vi "Double FFT Mesurament (Control - Init Wave&Window - Snapshot - DoubleFFT - Latency - Low Freq - FREQ LIN) RT Test.vi"() -> ()   [LabVIEW 2014]
uses:
  <vilib>/Platform/TimedLoop/XDataNode/timing_clust.ctl
  <vilib>/Platform/TimedLoop/XDataNode/nitl_modes.ctl
  <vilib>/Platform/TimedLoop/XDataNode/wakeup.ctl
  <vilib>/FPGAPlugInAG/sbRIO-9636/niLvFpga_Open_sbRIO-9636.vi
  <vilib>/rvi/interface/common/dynamic/niFpgaDynamicAddResources.vi
  <vilib>/Utility/error.llb/Error Cluster From Error Code.vi
  <vilib>/rvi/errors/niLvFpgaAdjustHostInterfaceError.vi
  <vilib>/rvi/interface/common/niFpgaWaitOnOcc.vi
  <vilib>/FPGAPlugInAG/Dynamic/niLvFpga_Run_Dynamic.vi
  <vilib>/FPGAPlugInAG/Dynamic/niLvFpga_Abort_Dynamic.vi
  <vilib>/FPGAPlugInAG/Dynamic/niLvFpga_Reset_Dynamic.vi
  <vilib>/FPGAPlugInAG/Dynamic/niLvFpga_Close_Dynamic.vi
  <vilib>/rvi/interface/nirviOpenFPGA/nirviOpenFPGA.xnode
  FPGA Bitfiles/LaserDistanceSen_FPGATarget_DoubleFFTMesuram_744PzgZsl5A.lvbitx
  FPGA Target/Test VIs/Double FFT Mesurament (Control - Init Wave&Window - Snapshot - DoubleFFT - Latency - Low Freq) test.vi
  <vilib>/rvi/interface/nirviReadWriteControl/nirviReadWriteControl.xnode
  <vilib>/rvi/interface/nirviMethod/nirviMethod.xnode
  <vilib>/Platform/TimedLoop/XDataNode/XDataNode.xnode
  <vilib>/rvi/interface/nirviCloseFPGA/nirviCloseFPGA.xnode
  <vilib>/FPGAPlugInAG/Dynamic/niLvFpga_ConfigureFifo_Dynamic.vi
  <vilib>/rvi/errors/niLvFpgaMergeErrorWithErrorCode.vi
  <vilib>/FPGAPlugInAG/Dynamic/niLvFpga_StartFifo_Dynamic.vi
  <vilib>/rvi/interface/Simulation/niFpgaSimulationCallBeginRW.vi
  <vilib>/FPGAPlugInAG/Dynamic/niLvFpga_ReadFifo_Dynamic.vi
  <vilib>/Platform/TimedLoop/XDataNode/XDNodeRunTimeDep.lvlib
  NiFpgaLv.dll
panel:
  in  "Acrive  Smooth":bool=TRUE
  out "Complete SkewTri":dbl[](graph)
  out "2) Tri edge":dbl[](graph)
  out "1) Tri edge":dbl[](graph)
  out "1) Ext Mean Freq Curve":dbl[](graph)
  out "2) Ext Mean Freq Curve":dbl[](graph)
  out "2) Mean Freq Curve":dbl[](graph)
  out "1) Mean Freq Curve":dbl[](graph)
  out "2) Freq curve":dbl[](graph)
  out "1) Freq curve":dbl[](graph)
  in  "FFT Sliding Win Size":i32=128
  out "1) SmoothSubSig":dbl[](graph)
  out "2) SmoothSubSig":dbl[](graph)
  in  "Acrive Fit":bool=TRUE
  in  "Poly Order":i32=3
  in  "Side points":i32=13
  in  "Poly Grade":dbl=5.0
  out "2) Signal&Fit 2":dbl[][](graph)
  out "1) Signal&Fit":dbl[][](graph)
  in  "tieni premuto per":i32=1
  out "Current Sig lin":i32
  in  "Acrive Linearization":bool
  in  "# Measurements for Linearization":i32=10
  in  "stop":bool
  out "maxbin_secondFFT":i32
  out "maxbin_firstFFT":i32
  out "f_rise":dbl
  out "f_fall":dbl
  out "f_mean":dbl
  out "Velocity (m/s)":dbl
  out "Distance (m)":dbl
  in  "Initial Latency points":u32(slide)=28 scale=0.0..1249.0
  out "Second FFT (bin)":dbl[](graph)
  out "Second Signal (points) - Rising Triangular":dbl[](graph)
  out "First FFT (bin)":dbl[](graph)
  out "First Signal (points) - Falling Triangular":dbl[](graph)
  in  "Snapshot":bool
  in  "Windowing":T1(ring)
  in  "first bin":i32=5
  in  "last bin":i32=255
  in  "lower limit 2":u32(slide)=738 scale=625.0..738.0
  in  "lower limit 1":u32(slide)=113 scale=0.0..113.0
  # "WARNING:\nOnce pressed wait untill the end of operation"
  # "OFFLINE parameters"
  # "Max Detection FFT bin range"
  # "ONLINE parameters"
  # "Se la sottrazione del fondo non è eseguita su FPGA.\n Attivarla per eseguirla lato RT"
  # "Smoothing (S-G Params)"
  # "Fitting"
  # "ONLY POWER OF 2"
  # "Min: 2 Max: 256 (2, 4, 8, 16, 32, 64, 128, 256)"
  # "LINEARIZATION FINAL RESULTS"
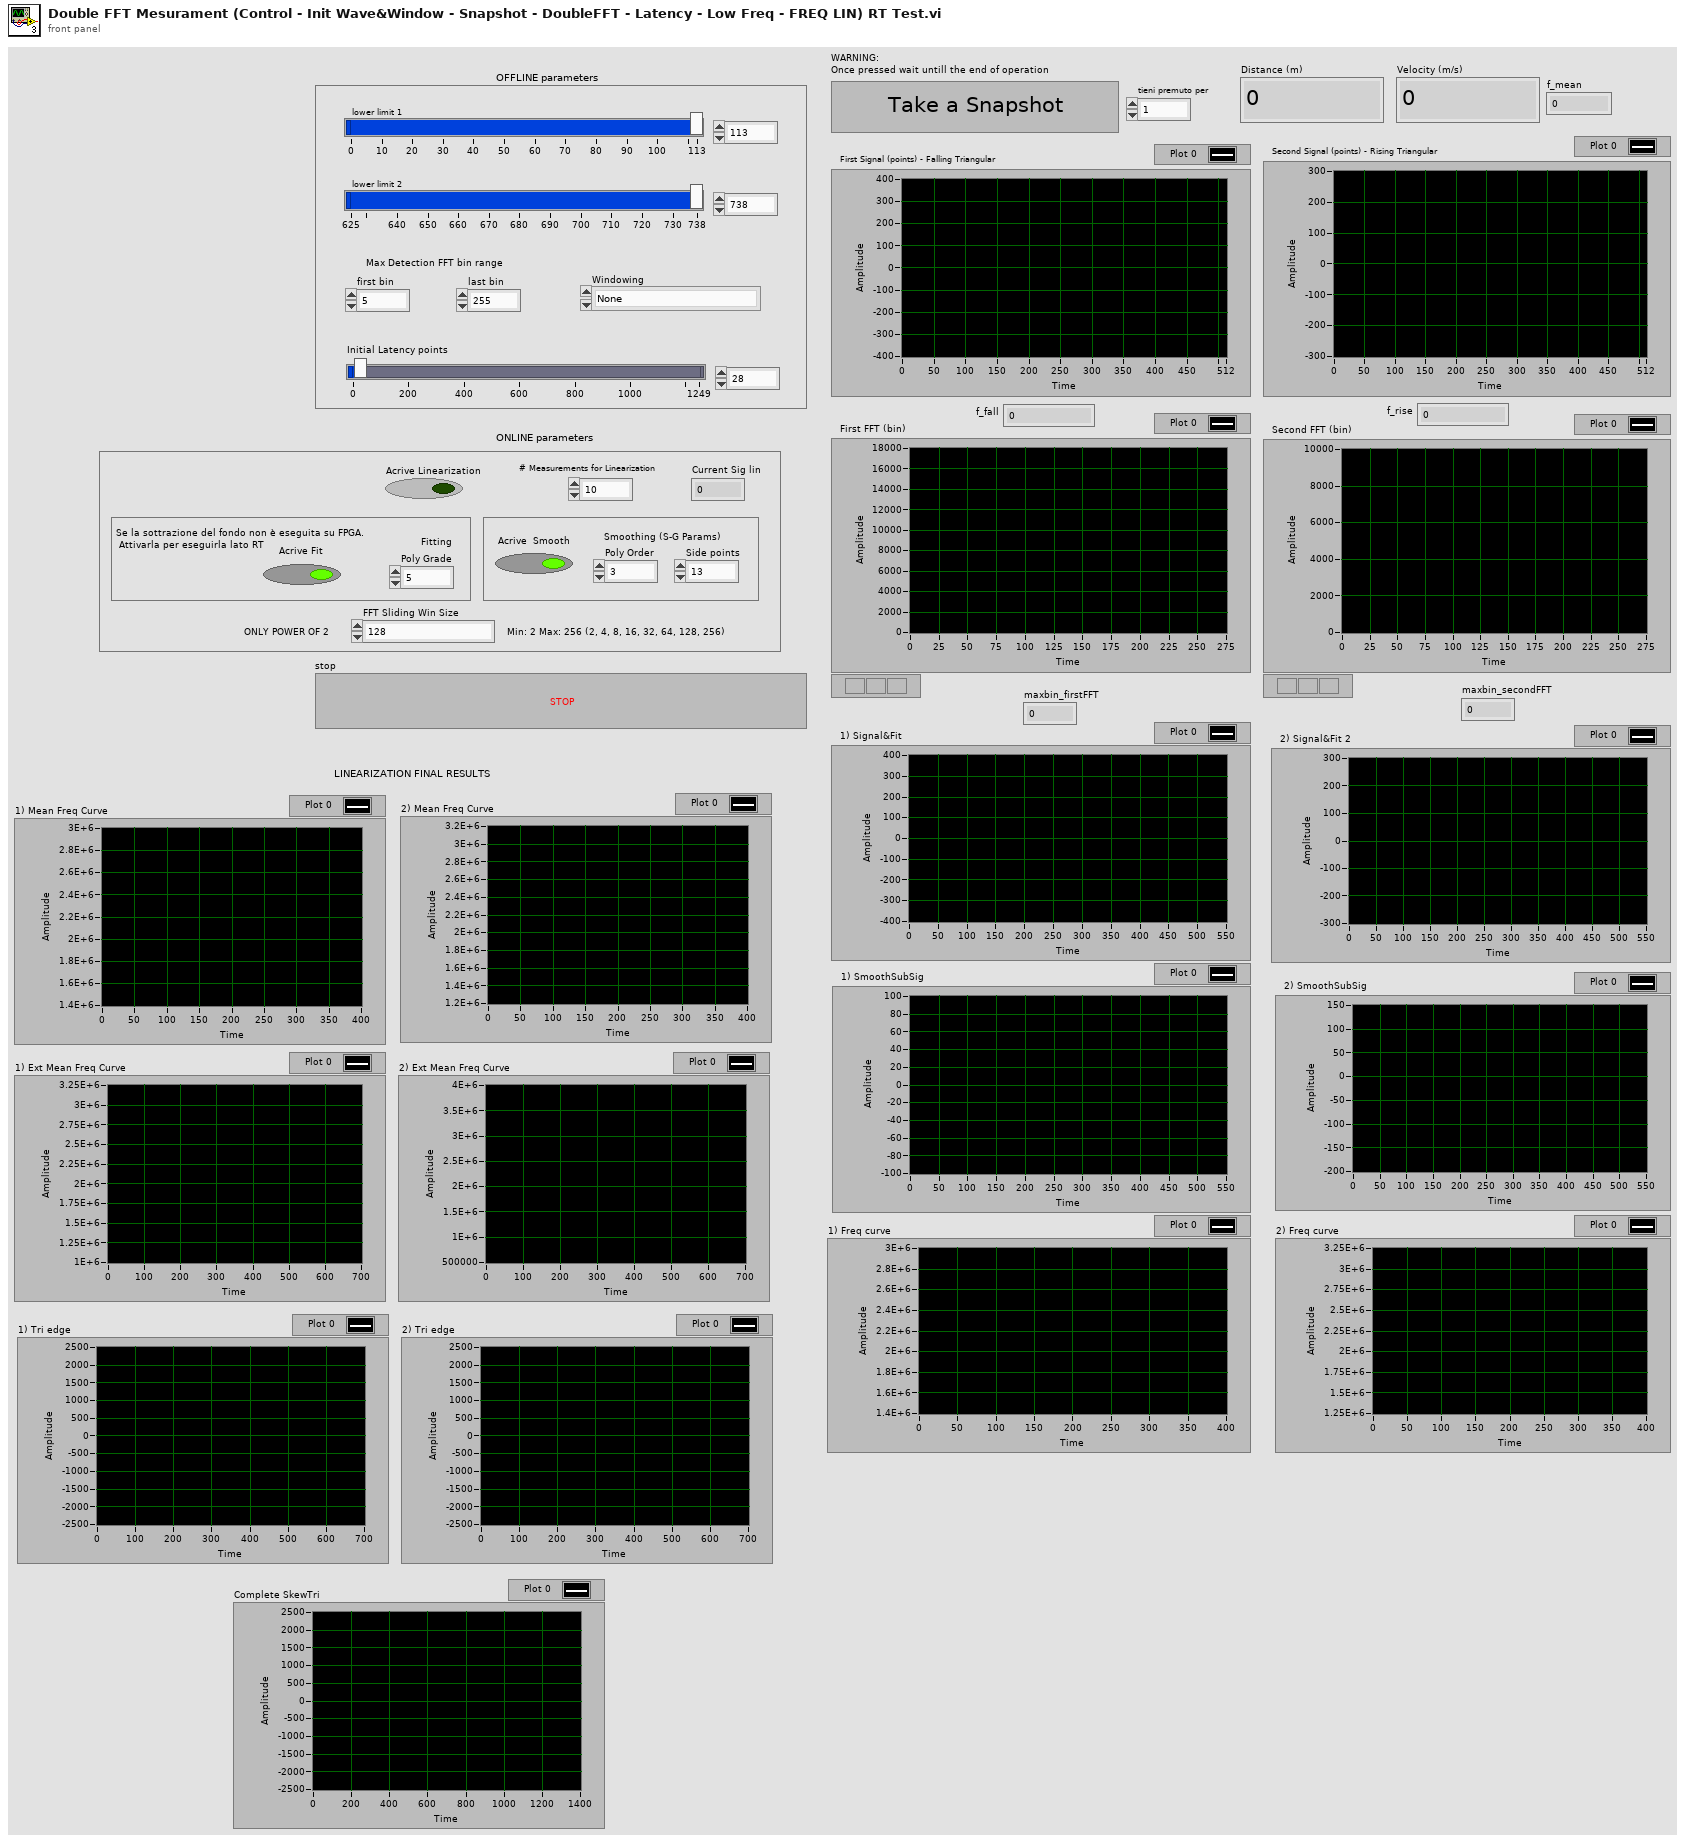
[diagram p1: front panel]
types:
  T1 = enum16{"None", "Hanning", "Hamming", "Blackman", "Blackman-Harris"}
  T2 = typedef "XDNodeRunTimeDep.lvlib/timing_clust.ctl" = cluster{"Expected End [f-1]":u64, "Actual End [f-1]":u64, "Finished Late? [f-1]":bool, "Expected End [i-1]":u64, "Actual End [i-1]":u64, "Finished Late? [i-1]":bool, "Expected Start [i]":u64, "Actual Start [i]":u64, "Expected Start [f]":u64, "Actual Start [f]":u64, "Source Name":string, "Structure Name":string, "Period":i64, "Deadline":i64, "Offset":i64, "Start":i64, "Priority":i32, "Timeout":i32, "Mode":T3, "Wakeup Reason":T4, "Error":errorcluster, "Source Type":string, "Secondary Source Type":string, "Global End Time":u64, "Global Start Time":u64, "Frame Duration":u64, "Iteration Duration":u64, "Assigned CPU":i32, "I/O Scan Engine Mode":u32}
  T3 = typedef "XDNodeRunTimeDep.lvlib/nitl_modes.ctl" = enum32{"No Change", "Process missed periods, maintain original phase", "Discard missed periods, maintain original phase", "Process missed periods, ignore original phase", "Discard missed periods, ignore original phase"}
  T4 = typedef "XDNodeRunTimeDep.lvlib/wakeup.ctl" = enum32{"Normal", "Aborted", "Asynchronous wakeup", "Timing source error", "Timed loop error", "Timeout"}
  T5 = typedef "NI_Matrix.lvlib/RealMatrix.ctl" = dbl[][]
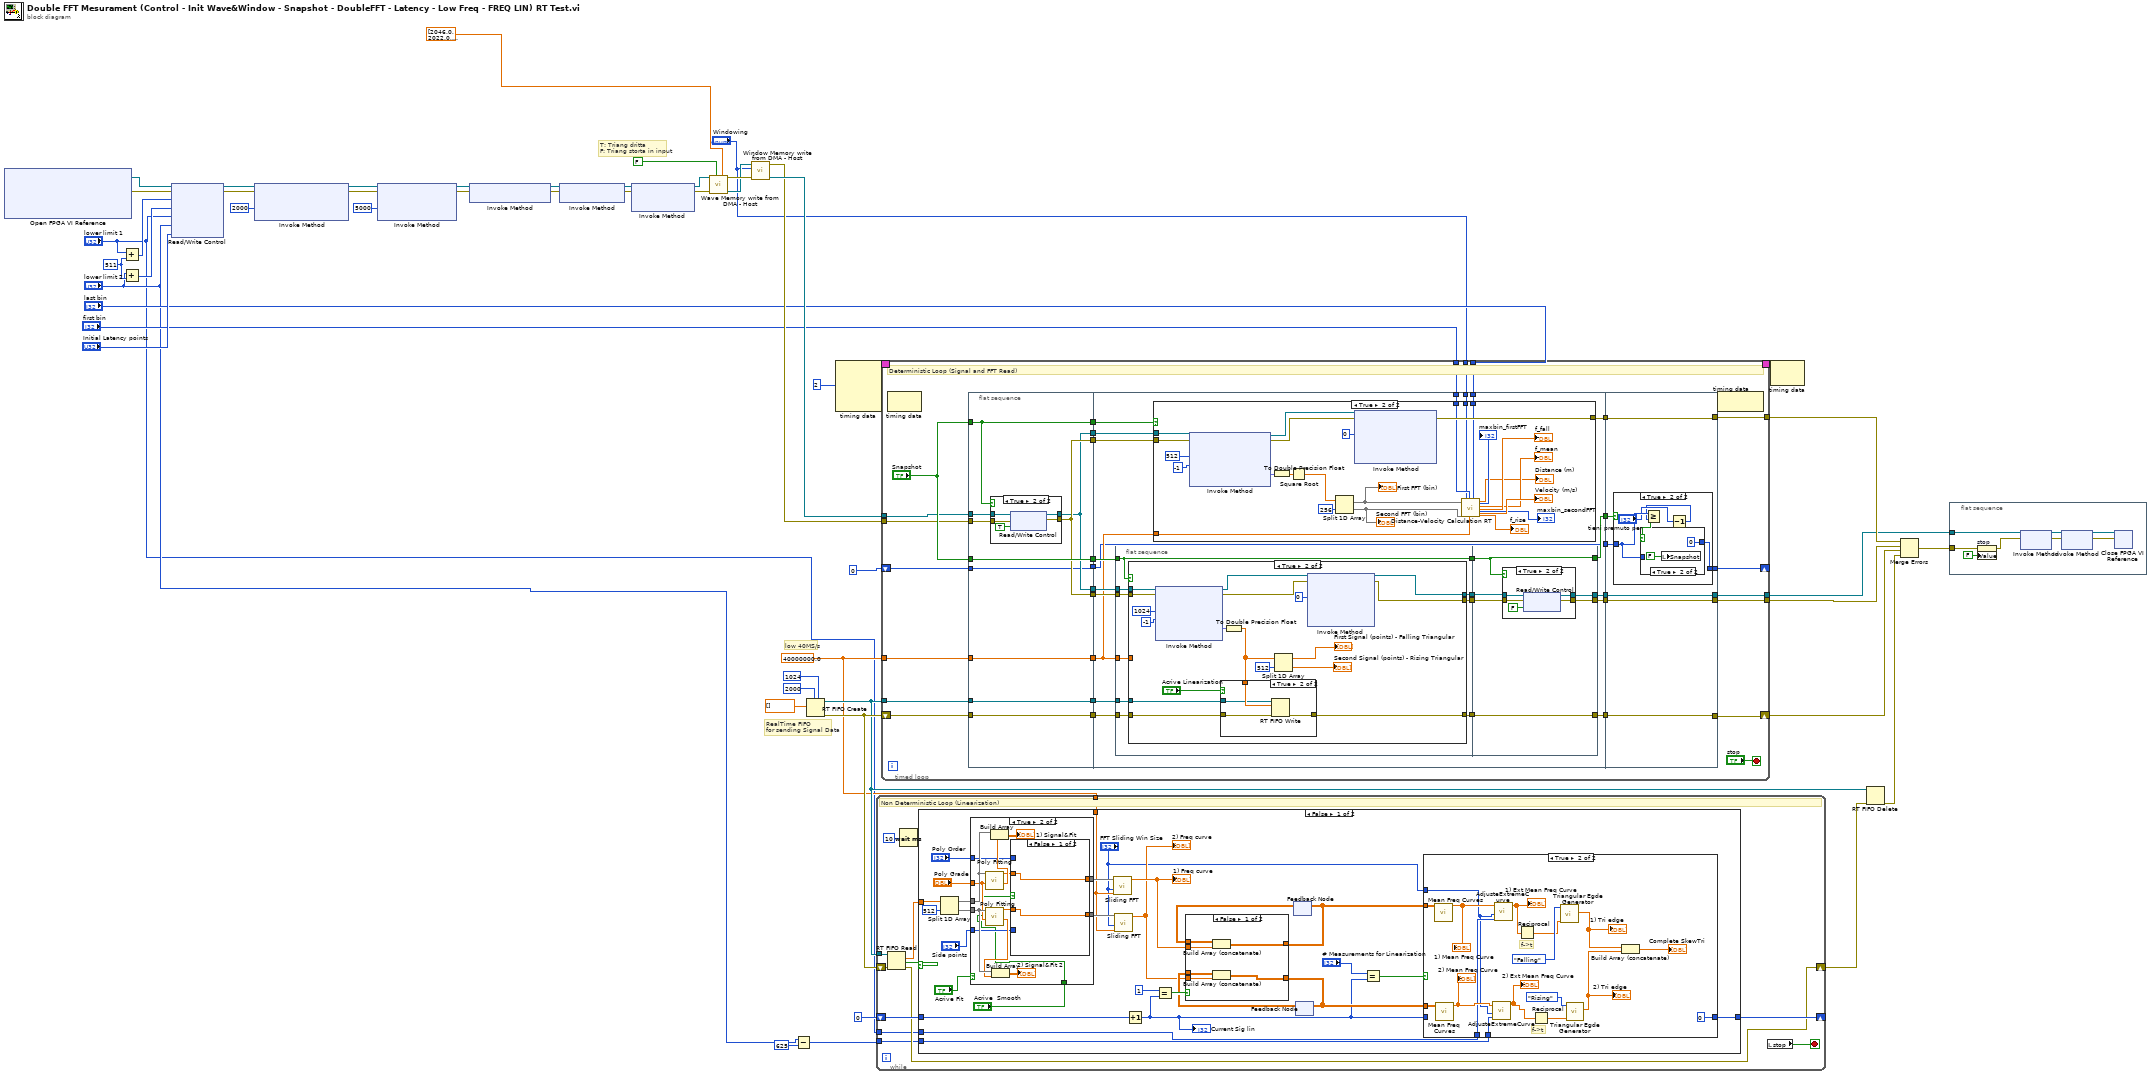
[diagram p0: block diagram]
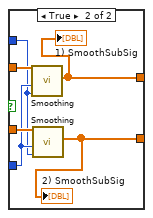
[diagram p3: hidden frame]
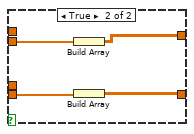
[diagram p5: hidden frame]
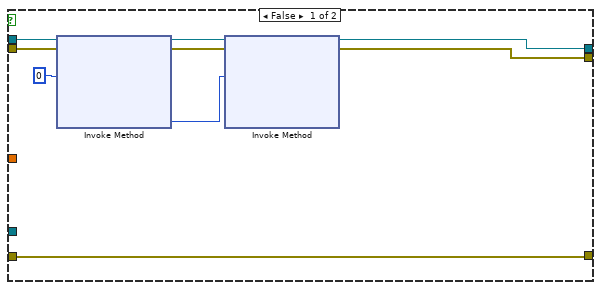
[diagram p8: hidden frame]
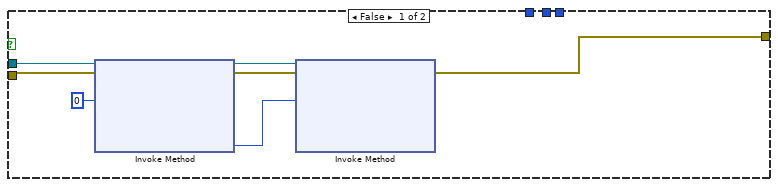
[diagram p11: hidden frame]
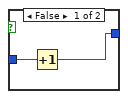
[diagram p13: hidden frame]
diagram:
  w49 = u32 511 ("y")
  w4 = 40000000.0 ("Sample Rate (S/s)")
  # "T: Triang dritta\nF: Triang storta in input"
  # "RealTime FIFO \nfor sending Signal Data"
  # "low 40MS/s"
  n1 = xnode "Open FPGA VI Reference"() -> ("FPGA VI Reference Out"=w48:refnum<k20>, "error out"=w47:errorcluster)  [unwired: 2 in]
  n2 = Add(x="lower limit 1", y=w49) -> (x+y=w51:u32)
  n3 = Add(x="lower limit 2", y=w49) -> (x+y=w50:u32)
  n4 = xnode "Read/Write Control"("FPGA VI Reference In"=w48, "error in"=w47, "upper limit 1"=w51, "upper limit 2"=w50, "lower limit 1"="lower limit 1", "lower limit 2"="lower limit 2", "Latency points"="Initial Latency points") -> ("FPGA VI Reference Out"=w44:refnum<k20>, "error out"=w43:errorcluster)
  n5 = xnode "Invoke Method"("FPGA VI Reference In"=w44, "error in"=w43, "Requested Depth"=u32 2000) -> ("FPGA VI Reference Out"=w22:refnum<k20>, "error out"=w23:errorcluster)  [unwired: 1 out]
  n6 = xnode "Invoke Method"("FPGA VI Reference In"=w22, "error in"=w23, "Requested Depth"=u32 5000) -> ("FPGA VI Reference Out"=w36:refnum<k20>, "error out"=w37:errorcluster)  [unwired: 1 out]
  n7 = xnode "Invoke Method"("FPGA VI Reference In"=w36, "error in"=w37) -> ("FPGA VI Reference Out"=w20:refnum<k20>, "error out"=w21:errorcluster)
  n8 = xnode "Invoke Method"("FPGA VI Reference In"=w20, "error in"=w21) -> ("FPGA VI Reference Out"=w34:refnum<k20>, "error out"=w35:errorcluster)
  n9 = xnode "Invoke Method"("FPGA VI Reference In"=w34, "error in"=w35) -> ("FPGA VI Reference Out"=w40:refnum<k20>, "error out"=w39:errorcluster)  [unwired: 1 in]
  n10 = call "Wave Memory write from DMA - Host.vi"("Custom Triangular Signal (fal-ris)"=dbl[] [2046.0, 2022.0, 1999.0, 1975.0, 1952.0, 1928.0, 1905.0, 1882.0, 1860.0, 1837.0, 1815.0, 1793.0, 1771.0, 1749.0, 1728.0, 1706.0, 1685.0, 1664.0, 1643.0, 1622.0, 1602.0, 1581.0, 1561.0, 1541.0, 1521.0, 1501.0, 1482.0, 1462.0, 1443.0, 1424.0, 1405.0, 1386.0, 1367.0, 1348.0, 1330.0, 1312.0, 1293.0, 1275.0, 1257.0, 1240.0, 1222.0, 1204.0, 1187.0, 1170.0, 1153.0, 1136.0, 1119.0, 1102.0, 1085.0, 1069.0, 1052.0, 1036.0, 1020.0, 1004.0, 988.0, 972.0, 956.0, 940.0, 925.0, 910.0, 894.0, 879.0, 864.0, 849.0, 834.0, 819.0, 804.0, 790.0, 775.0, 761.0, 747.0, 732.0, 718.0, 704.0, 690.0, 676.0, 663.0, 649.0, 635.0, 622.0, 608.0, 595.0, 582.0, 569.0, 555.0, 542.0, 530.0, 517.0, 504.0, 491.0, 479.0, 466.0, 454.0, 441.0, 429.0, 417.0, 405.0, 393.0, 381.0, 369.0, 357.0, 345.0, 333.0, 322.0, 310.0, 299.0, 287.0, 276.0, 265.0, 253.0, 242.0, 231.0, 220.0, 209.0, 198.0, 187.0, 176.0, 166.0, 155.0, 144.0, 134.0, 123.0, 113.0, 103.0, 92.0, 82.0, 72.0, 62.0, 52.0, 42.0, 32.0, 22.0, 12.0, 2.0, -8.0, -17.0, -27.0, -37.0, -46.0, -56.0, -65.0, -75.0, -84.0, -93.0, -102.0, -112.0, -121.0, -130.0, -139.0, -148.0, -157.0, -166.0, -175.0, -184.0, -192.0, -201.0, -210.0, -218.0, -227.0, -235.0, -244.0, -252.0, -261.0, -269.0, -278.0, -289.0, -298.0, -306.0, -314.0, -323.0, -331.0, -339.0, -348.0, -356.0, -364.0, -372.0, -380.0, -388.0, -396.0, -404.0, -412.0, -420.0, -428.0, -436.0, -443.0, -451.0, -458.0, -466.0, -473.0, -481.0, -488.0, -495.0, -502.0, -509.0, -516.0, -523.0, -530.0, -536.0, -543.0, -550.0, -562.0, -568.0, -575.0, -587.0, -595.0, -602.0, -608.0, -614.0, -621.0, -627.0, -637.0, -643.0, -650.0, -656.0, -666.0, -672.0, -681.0, -689.0, -696.0, -702.0, -707.0, -713.0, -719.0, -725.0, -730.0, -736.0, -742.0, -747.0, -753.0, -758.0, -764.0, -769.0, -775.0, -780.0, -786.0, -791.0, -797.0, -802.0, -807.0, -813.0, -818.0, -823.0, -828.0, -833.0, -839.0, -844.0, -849.0, -854.0, -859.0, -864.0, -870.0, -875.0, -880.0, -885.0, -890.0, -895.0, -900.0, -905.0, -910.0, -915.0, -919.0, -924.0, -929.0, -934.0, -940.0, -945.0, -950.0, -954.0, -959.0, -964.0, -969.0, -974.0, -978.0, -984.0, -989.0, -994.0, -1000.0, -1004.0, -1009.0, -1013.0, -1019.0, -1023.0, -1027.0, -1032.0, -1037.0, -1042.0, -1047.0, -1052.0, -1056.0, -1060.0, -1065.0, -1069.0, -1073.0, -1077.0, -1081.0, -1085.0, -1089.0, -1093.0, -1097.0, -1101.0, -1105.0, -1109.0, -1113.0, -1116.0, -1120.0, -1124.0, -1128.0, -1131.0, -1135.0, -1139.0, -1142.0, -1146.0, -1150.0, -1153.0, -1157.0, -1161.0, -1164.0, -1168.0, -1171.0, -1175.0, -1178.0, -1182.0, -1185.0, -1189.0, -1192.0, -1196.0, -1199.0, -1203.0, -1206.0, -1210.0, -1213.0, -1217.0, -1220.0, -1224.0, -1227.0, -1231.0, -1234.0, -1237.0, -1241.0, -1244.0, -1248.0, -1251.0, -1255.0, -1258.0, -1262.0, -1265.0, -1268.0, -1272.0, -1275.0, -1279.0, -1282.0, -1286.0, -1289.0, -1292.0, -1296.0, -1299.0, -1303.0, -1306.0, -1310.0, -1313.0, -1316.0, -1320.0, -1323.0, -1327.0, -1330.0, -1334.0, -1337.0, -1340.0, -1344.0, -1347.0, -1351.0, -1354.0, -1357.0, -1361.0, -1364.0, -1368.0, -1371.0, -1374.0, -1377.0, -1381.0, -1384.0, -1387.0, -1390.0, -1394.0, -1397.0, -1400.0, -1404.0, -1407.0, -1410.0, -1413.0, -1417.0, -1420.0, -1423.0, -1426.0, -1429.0, -1432.0, -1435.0, -1438.0, -1441.0, -1444.0, -1448.0, -1451.0, -1454.0, -1457.0, -1460.0, -1463.0, -1466.0, -1469.0, -1472.0, -1475.0, -1478.0, -1481.0, -1484.0, -1487.0, -1490.0, -1493.0, -1496.0, -1499.0, -1502.0, -1505.0, -1508.0, -1511.0, -1515.0, -1517.0, -1520.0, -1523.0, -1526.0, -1529.0, -1533.0, -1536.0, -1539.0, -1542.0, -1544.0, -1547.0, -1550.0, -1553.0, -1556.0, -1559.0, -1562.0, -1565.0, -1568.0, -1570.0, -1573.0, -1576.0, -1579.0, -1582.0, -1585.0, -1587.0, -1590.0, -1593.0, -1596.0, -1599.0, -1602.0, -1604.0, -1607.0, -1610.0, -1613.0, -1616.0, -1618.0, -1621.0, -1624.0, -1627.0, -1630.0, -1632.0, -1635.0, -1638.0, -1641.0, -1644.0, -1646.0, -1649.0, -1652.0, -1655.0, -1657.0, -1660.0, -1663.0, -1666.0, -1668.0, -1671.0, -1674.0, -1677.0, -1679.0, -1682.0, -1685.0, -1688.0, -1690.0, -1693.0, -1696.0, -1699.0, -1701.0, -1704.0, -1707.0, -1709.0, -1712.0, -1715.0, -1718.0, -1720.0, -1723.0, -1726.0, -1728.0, -1731.0, -1734.0, -1736.0, -1739.0, -1742.0, -1744.0, -1747.0, -1750.0, -1752.0, -1755.0, -1758.0, -1760.0, -1763.0, -1766.0, -1768.0, -1771.0, -1774.0, -1776.0, -1779.0, -1782.0, -1784.0, -1787.0, -1790.0, -1792.0, -1795.0, -1797.0, -1800.0, -1803.0, -1805.0, -1808.0, -1811.0, -1813.0, -1816.0, -1818.0, -1821.0, -1824.0, -1826.0, -1829.0, -1831.0, -1834.0, -1837.0, -1839.0, -1842.0, -1844.0, -1847.0, -1850.0, -1852.0, -1855.0, -1857.0, -1860.0, -1862.0, -1865.0, -1868.0, -1870.0, -1873.0, -1875.0, -1878.0, -1880.0, -1883.0, -1885.0, -1888.0, -1891.0, -1893.0, -1896.0, -1898.0, -1901.0, -1903.0, -1906.0, -1908.0, -1911.0, -1913.0, -1916.0, -1918.0, -1921.0, -1923.0, -1926.0, -1928.0, -1931.0, -1933.0, -1936.0, -1938.0, -1941.0, -1943.0, -1946.0, -1948.0, -1951.0, -1953.0, -1956.0, -1958.0, -1961.0, -1963.0, -1966.0, -1968.0, -1971.0, -1973.0, -1976.0, -1978.0, -1981.0, -1983.0, -1985.0, -1988.0, -1990.0, -1993.0, -1995.0, -1998.0, -2000.0, -2003.0, -2005.0, -2007.0, -2010.0, -2012.0, -2015.0, -2017.0, -2020.0, -2022.0, -2024.0, -2027.0, -2029.0, -2032.0, -2034.0, -2036.0, -2039.0, -2041.0, -2044.0, -2046.0, -2048.0, -2048.0, -2013.0, -1979.0, -1945.0, -1911.0, -1879.0, -1847.0, -1815.0, -1784.0, -1754.0, -1724.0, -1694.0, -1666.0, -1637.0, -1609.0, -1582.0, -1555.0, -1529.0, -1503.0, -1477.0, -1452.0, -1427.0, -1403.0, -1379.0, -1355.0, -1332.0, -1309.0, -1286.0, -1264.0, -1242.0, -1221.0, -1200.0, -1179.0, -1158.0, -1138.0, -1118.0, -1098.0, -1079.0, -1060.0, -1041.0, -1022.0, -1004.0, -986.0, -968.0, -950.0, -933.0, -916.0, -899.0, -882.0, -866.0, -849.0, -833.0, -818.0, -802.0, -786.0, -771.0, -756.0, -741.0, -727.0, -712.0, -698.0, -684.0, -670.0, -656.0, -642.0, -629.0, -616.0, -602.0, -589.0, -576.0, -564.0, -551.0, -539.0, -527.0, -514.0, -502.0, -491.0, -479.0, -467.0, -456.0, -444.0, -433.0, -422.0, -411.0, -400.0, -389.0, -379.0, -368.0, -358.0, -348.0, -337.0, -327.0, -317.0, -307.0, -298.0, -288.0, -278.0, -269.0, -259.0, -250.0, -241.0, -232.0, -223.0, -214.0, -205.0, -196.0, -187.0, -179.0, -170.0, -162.0, -154.0, -145.0, -137.0, -129.0, -121.0, -113.0, -105.0, -97.0, -89.0, -82.0, -74.0, -66.0, -59.0, -51.0, -44.0, -37.0, -30.0, -22.0, -15.0, -8.0, -1.0, 6.0, 13.0, 19.0, 26.0, 33.0, 40.0, 46.0, 53.0, 59.0, 66.0, 72.0, 78.0, 85.0, 91.0, 97.0, 103.0, 109.0, 115.0, 121.0, 127.0, 133.0, 139.0, 145.0, 150.0, 156.0, 162.0, 167.0, 173.0, 178.0, 184.0, 189.0, 195.0, 200.0, 205.0, 211.0, 216.0, 221.0, 226.0, 231.0, 232.0, 238.0, 243.0, 249.0, 254.0, 259.0, 265.0, 270.0, 276.0, 281.0, 281.0, 283.0, 289.0, 294.0, 288.0, 273.0, 276.0, 282.0, 288.0, 293.0, 296.0, 293.0, 295.0, 301.0, 307.0, 313.0, 309.0, 314.0, 314.0, 314.0, 319.0, 324.0, 328.0, 333.0, 338.0, 342.0, 347.0, 351.0, 356.0, 360.0, 365.0, 369.0, 374.0, 378.0, 383.0, 387.0, 392.0, 396.0, 401.0, 402.0, 407.0, 412.0, 413.0, 418.0, 424.0, 429.0, 431.0, 437.0, 443.0, 448.0, 447.0, 448.0, 451.0, 455.0, 461.0, 464.0, 459.0, 465.0, 470.0, 474.0, 480.0, 484.0, 490.0, 490.0, 496.0, 502.0, 508.0, 513.0, 519.0, 525.0, 530.0, 536.0, 536.0, 541.0, 547.0, 552.0, 558.0, 563.0, 569.0, 574.0, 579.0, 584.0, 590.0, 595.0, 600.0, 605.0, 611.0, 616.0, 621.0, 627.0, 632.0, 637.0, 642.0, 648.0, 653.0, 659.0, 664.0, 669.0, 675.0, 680.0, 686.0, 691.0, 697.0, 702.0, 708.0, 714.0, 719.0, 725.0, 725.0, 731.0, 737.0, 744.0, 747.0, 753.0, 759.0, 766.0, 772.0, 777.0, 784.0, 790.0, 798.0, 805.0, 811.0, 816.0, 815.0, 821.0, 823.0, 826.0, 831.0, 837.0, 842.0, 840.0, 843.0, 845.0, 851.0, 856.0, 861.0, 866.0, 871.0, 869.0, 869.0, 873.0, 878.0, 883.0, 887.0, 892.0, 897.0, 901.0, 906.0, 906.0, 910.0, 914.0, 918.0, 922.0, 926.0, 930.0, 934.0, 937.0, 941.0, 945.0, 949.0, 953.0, 956.0, 960.0, 964.0, 968.0, 972.0, 976.0, 980.0, 984.0, 988.0, 992.0, 996.0, 1000.0, 1004.0, 1008.0, 1012.0, 1016.0, 1021.0, 1026.0, 1031.0, 1036.0, 1041.0, 1045.0, 1050.0, 1055.0, 1054.0, 1059.0, 1061.0, 1060.0, 1065.0, 1070.0, 1075.0, 1080.0, 1083.0, 1086.0, 1091.0, 1094.0, 1097.0, 1098.0, 1101.0, 1105.0, 1110.0, 1113.0, 1117.0, 1122.0, 1126.0, 1131.0, 1136.0, 1139.0, 1144.0, 1148.0, 1153.0, 1158.0, 1163.0, 1167.0, 1172.0, 1177.0, 1182.0, 1186.0, 1191.0, 1196.0, 1201.0, 1206.0, 1210.0, 1215.0, 1220.0, 1225.0, 1230.0, 1235.0, 1240.0, 1245.0, 1250.0, 1255.0, 1260.0, 1265.0, 1270.0, 1275.0, 1280.0, 1285.0, 1290.0, 1295.0, 1301.0, 1306.0, 1311.0, 1316.0, 1321.0, 1326.0, 1331.0, 1335.0, 1340.0, 1345.0, 1350.0, 1355.0, 1359.0, 1364.0, 1369.0, 1373.0, 1378.0, 1382.0, 1387.0, 1391.0, 1396.0, 1400.0, 1404.0, 1408.0, 1413.0, 1417.0, 1421.0, 1425.0, 1429.0, 1434.0, 1438.0, 1442.0, 1446.0, 1450.0, 1454.0, 1459.0, 1463.0, 1467.0, 1471.0, 1475.0, 1479.0, 1483.0, 1487.0, 1491.0, 1495.0, 1499.0, 1503.0, 1507.0, 1511.0, 1515.0, 1519.0, 1523.0, 1527.0, 1531.0, 1535.0, 1539.0, 1543.0, 1547.0, 1551.0, 1555.0, 1559.0, 1563.0, 1567.0, 1571.0, 1574.0, 1578.0, 1582.0, 1586.0, 1590.0, 1594.0, 1598.0, 1602.0, 1605.0, 1609.0, 1613.0, 1617.0, 1621.0, 1624.0, 1628.0, 1632.0, 1636.0, 1639.0, 1643.0, 1647.0, 1651.0, 1654.0, 1658.0, 1662.0, 1666.0, 1669.0, 1673.0, 1677.0, 1680.0, 1684.0, 1688.0, 1691.0, 1695.0, 1699.0, 1702.0, 1706.0, 1710.0, 1713.0, 1717.0, 1720.0, 1724.0, 1728.0, 1731.0, 1735.0, 1738.0, 1742.0, 1745.0, 1749.0, 1753.0, 1756.0, 1760.0, 1763.0, 1767.0, 1770.0, 1774.0, 1777.0, 1781.0, 1784.0, 1788.0, 1791.0, 1795.0, 1798.0, 1802.0, 1805.0, 1808.0, 1812.0, 1815.0, 1819.0, 1822.0, 1826.0, 1829.0, 1832.0, 1836.0, 1839.0, 1842.0, 1846.0, 1849.0, 1853.0, 1856.0, 1859.0, 1863.0, 1866.0, 1869.0, 1873.0, 1876.0, 1879.0, 1883.0, 1886.0, 1889.0, 1892.0, 1896.0, 1899.0, 1902.0, 1906.0, 1909.0, 1912.0, 1915.0, 1918.0, 1922.0, 1925.0, 1928.0, 1931.0, 1935.0, 1938.0, 1941.0, 1944.0, 1947.0, 1951.0, 1954.0, 1957.0, 1960.0, 1963.0, 1966.0, 1970.0, 1973.0, 1976.0, 1979.0, 1982.0, 1985.0, 1988.0, 1991.0, 1995.0, 1998.0, 2001.0, 2004.0, 2007.0, 2010.0, 2013.0, 2016.0, 2019.0, 2022.0, 2025.0, 2028.0, 2031.0, 2034.0, 2037.0, 2040.0, 2043.0, 2047.0] ("Complete SkewTri"), "Triangolo dritto?"=FALSE, "error in"=w39, "FPGA VI Reference In"=w40) -> ("FPGA VI Reference Out"=w25:refnum<k20>, "error out"=w38:errorcluster)  [unwired: 5 in, 1 out]
  n11 = call "Window Memory write from DMA - Host.vi"("error in"=w38, "Enum"="Windowing", "FPGA VI Reference In"=w25) -> ("FPGA VI Reference Out"=w46:refnum<k20>, "error out"=w45:errorcluster)  [unwired: 5 in, 2 out]
  n12 = Subtract(x="lower limit 2", y=u32 625) -> (x-y=w6:u32)
  n13 = RT FIFO Create(1:dbl[] [] ("double precision float"), 4:u32 2000 ("size (10)"), 6:u32 1024 ("elements in array (1)")) -> (8:w12:refnum<k33>, 11:w14:errorcluster)  [unwired: 5 in, 1 out]
  n14 = node-c288(i64 2 ("Period")) -> (w33:T2)  [unwired: 3 in]
  n15 = while {
    shift-right: [w55] -> w11
    shift-left: w14 -> [w57]
    tunnel: w12 -> [w62]
    shift-right: [w56] -> _
    shift-left: 0 -> [w60]
    tunnel: "lower limit 1" -> [w52]
    tunnel: w6 -> [w53]
    tunnel: w4 -> [w54]
    stop <- w61 stop-if-true
    # "Non Deterministic Loop (Linearization)"
    n16 = RT FIFO Read(0:w62, 3:w57) -> (9:w59:dbl[], 10:w58:bool, 11:w55:errorcluster)  [unwired: 2 in, 2 out]
    n17 = Wait (ms)(milliseconds to wait=u32 10 ("millisecond multiple")) -> ()  [unwired: 1 out]
    n18 = case shown="False" w58 {
      tunnel: w60 -> [w91 w144]
      tunnel: [w80 w144] -> w56
      tunnel: w59 -> [w89 _]
      tunnel: w54 -> [w70 _]
      tunnel: w53 -> [w67 _]
      tunnel: w52 -> [w66 _]
      frame False {
        n19 = Split 1D Array(array=w89, index=512) -> (first subarray=w78:dbl[], second subarray=w77:dbl[])
        n20 = case shown="True" "Acrive Fit" {
          tunnel: w78 -> [w93 w107]
          tunnel: w77 -> [w92 w103]
          tunnel: "Poly Grade" -> [_ w99]
          tunnel: "Side points" -> [_ w98]
          tunnel: "Poly Order" -> [_ w97]
          tunnel: [w92 w96] -> w71
          tunnel: [w93 w94] -> w72
          tunnel: "Acrive  Smooth" -> [_ w95]
          frame False {
          }
          frame True {
            n21 = call "Poly Fitting.vi"("Poly Grade"=w99, "Signal"=w107) -> ("Poly Signal"=w106:dbl[], "SubtractedSignal"=w101:dbl[])  [unwired: 8 in]
            n22 = call "Poly Fitting.vi"("Poly Grade"=w99, "Signal"=w103) -> ("Poly Signal"=w102:dbl[], "SubtractedSignal"=w100:dbl[])  [unwired: 8 in]
            n23 = Build Array(w107, w106) -> (→"1) Signal&Fit":dbl[][])
            n24 = Build Array(w103, w102) -> (→"2) Signal&Fit 2":dbl[][])
            n25 = case shown="False" w95 {
              tunnel: w101 -> [w109 w115]
              tunnel: w100 -> [w108 w114]
              tunnel: w98 -> [_ w113]
              tunnel: w97 -> [_ w112]
              tunnel: [w108 w111] -> w96
              tunnel: [w109 w110] -> w94
              frame False {
              }
              frame True {
                n26 = call "Smoothing.vi"("polynomial order"=w112, "side points"=w113, "SubtractedSignal"=w115) -> ("SubSmoothSignal"=w110:dbl[])  [unwired: 8 in]
                "1) SmoothSubSig" <- w110
                n27 = call "Smoothing.vi"("polynomial order"=w112, "side points"=w113, "SubtractedSignal"=w114) -> ("SubSmoothSignal"=w111:dbl[])  [unwired: 8 in]
                "2) SmoothSubSig" <- w111
              }
            }
          }
        }
        n28 = call "Sliding FFT.vi"("Sample Freq"=w70, "FFT Win Size"="FFT Sliding Win Size", "SubSmoothSignal"=w72) -> ("Freq samples"=w69:dbl[])  [unwired: 7 in, 1 out]
        "1) Freq curve" <- w69
        n29 = call "Sliding FFT.vi"("Sample Freq"=w70, "FFT Win Size"="FFT Sliding Win Size", "SubSmoothSignal"=w71) -> ("Freq samples"=w68:dbl[])  [unwired: 7 in, 1 out]
        "2) Freq curve" <- w68
        n30 = Increment(x=w91) -> (x+1=w81:i32)
        "Current Sig lin" <- w81
        n31 = Equal?(x=1, y=w81) -> (x = y?=w87:bool)
        n32 = feedback #1() -> (w86:T5)  [unwired: 1 in]
        n33 = feedback #2() -> (w85:T5)  [unwired: 1 in]
        n34 = case shown="False" w87 {
          tunnel: w68 -> [w138 w141]
          tunnel: w69 -> [w139 w143]
          tunnel: [w137 w140] -> w82
          tunnel: [w136 w142] -> w83
          tunnel: w86 -> [w135 _]
          tunnel: w85 -> [w134 _]
          frame False {
            n35 = Build Array (concatenate)(w135, w139) -> (w136:T5)
            n36 = Build Array (concatenate)(w134, w138) -> (w137:T5)
          }
          frame True {
            n37 = Build Array(w143) -> (w142:T5)
            n38 = Build Array(w141) -> (w140:T5)
          }
        }
        n39 = feedback-in #1(w83) -> ()
        n40 = feedback-in #2(w82) -> ()
        n41 = Equal?(x="# Measurements for Linearization", y=w81) -> (x = y?=w79:bool)
        n42 = case shown="True" w79 {
          tunnel: w83 -> [_ w132]
          tunnel: w82 -> [_ w131]
          tunnel: w81 -> [w116 _]
          tunnel: [w116 0] -> w80
          tunnel: w67 -> [_ w122]
          tunnel: w66 -> [_ w119]
          tunnel: "FFT Sliding Win Size" -> [_ w118]
          frame False {
          }
          frame True {
            # "f->t"
            # "f->t"
            n43 = call "Mean Freq Curves.vi"("Set of Freq samples"=w132) -> ("Mean Freq Curve"=w123:dbl[])  [unwired: 10 in]
            "1) Mean Freq Curve" <- w123
            n44 = call "Mean Freq Curves.vi"("Set of Freq samples"=w131) -> ("Mean Freq Curve"=w120:dbl[])  [unwired: 10 in]
            "2) Mean Freq Curve" <- w120
            n45 = call "AdjusteExtremeCurve.vi"("Init Bins Discarded"=w122, "FFT Size Window"=w118, "Freq sample"=w120) -> ("Extended Freq Sample"=w121:dbl[])  [unwired: 8 in]
            "2) Ext Mean Freq Curve" <- w121
            n46 = call "AdjusteExtremeCurve.vi"("Init Bins Discarded"=w119, "FFT Size Window"=w118, "Freq sample"=w123) -> ("Extended Freq Sample"=w117:dbl[])  [unwired: 8 in]
            "1) Ext Mean Freq Curve" <- w117
            n47 = Reciprocal(x=w117) -> (1/x=w125:dbl[])
            n48 = Reciprocal(x=w121) -> (1/x=w124:dbl[])
            n49 = call "Triangular Egde Generator.vi"("Sample values"=w125, "Triangular edge"=enum16{"Rising", "Falling"}."Falling") -> ("Skew Triangular"=w128:dbl[])  [unwired: 9 in]
            "1) Tri edge" <- w128
            n50 = call "Triangular Egde Generator.vi"("Sample values"=w124, "Triangular edge"=enum16{"Rising", "Falling"}."Rising") -> ("Skew Triangular"=w127:dbl[])  [unwired: 9 in]
            "2) Tri edge" <- w127
            n51 = Build Array (concatenate)(w128, w127) -> (→"Complete SkewTri":dbl[])
          }
        }
      }
      frame True {
      }
    }
    n52 = local read "stop"() -> (w61:bool)
  }
  n53 = timed-loop {
    tunnel: w46 -> [w171]
    tunnel: w45 -> [w172]
    tunnel: [w174] -> w30
    tunnel: w4 -> [w176]
    tunnel: [w175] -> w29
    timing: w33 -> [_]
    timing-out: [_] -> w32
    tunnel: "first bin" -> [w160]
    tunnel: "last bin" -> [w159]
    tunnel: [w157] -> w24
    tunnel: "Windowing" -> [w155]
    shift-right: [w149] -> w15
    shift-left: w14 -> [w151]
    tunnel: w12 -> [w153]
    shift-right: [w145] -> _
    shift-left: 0 -> [w147]
    stop <- "stop" stop-if-true
    # "Deterministic Loop (Signal and FFT Read)"
    n54 = node-c288() -> ()  [unwired: 1 in, 1 out]
    n55 = flat-sequence {
      tunnel: w171 -> [w184]
      tunnel: w172 -> [w185]
      tunnel: "Snapshot" -> [w182]
      tunnel: "Snapshot" -> [w187]
      tunnel: w176 -> [w188]
      tunnel: [w186] -> w170
      tunnel: [w188] -> w169
      tunnel: [w187] -> w168
      tunnel: [w182] -> w167
      tunnel: [w186] -> w166
      tunnel: [w183] -> w165
      tunnel: [w183] -> w164
      tunnel: [w181] -> w154
      tunnel: w153 -> [w181]
      tunnel: [w180] -> w152
      tunnel: w151 -> [w180]
      tunnel: [w179] -> w148
      tunnel: w147 -> [w179]
      tunnel: w170 -> [w213]
      tunnel: w169 -> [w201]
      tunnel: w168 -> [w207]
      tunnel: w167 -> [w210]
      tunnel: w166 -> [w209]
      tunnel: w165 -> [w208]
      tunnel: w164 -> [w214]
      tunnel: [w212] -> w163
      tunnel: [w211] -> w162
      tunnel: [w206] -> w161
      tunnel: w160 -> [w205]
      tunnel: w159 -> [w204]
      tunnel: [w203] -> w156
      tunnel: w155 -> [w202]
      tunnel: w154 -> [w200]
      tunnel: w152 -> [w199]
      tunnel: [w197] -> w150
      tunnel: w148 -> [w196]
      tunnel: [w196] -> w146
      tunnel: [w309] -> w174
      tunnel: [w310] -> w175
      tunnel: w163 -> [w310]
      tunnel: w162 -> [w309]
      tunnel: w161 -> [w308]
      tunnel: [w307] -> w157
      tunnel: w156 -> [w307]
      tunnel: [w306] -> w149
      tunnel: w150 -> [w306]
      tunnel: w146 -> [w305]
      tunnel: [w304] -> w145
      frame #0 {
        n56 = case shown="True" w182 {
          tunnel: [w189 w194] -> w186
          tunnel: w185 -> [w189 w193]
          tunnel: w184 -> [w190 w192]
          tunnel: [w190 w191] -> w183
          frame False {
          }
          frame True {
            n57 = xnode "Read/Write Control"("FPGA VI Reference In"=w192, "error in"=w193, "snapshot"=TRUE) -> ("FPGA VI Reference Out"=w191:refnum<k20>, "error out"=w194:errorcluster)
          }
        }
      }
      frame #1 {
        n58 = flat-sequence {
          tunnel: w214 -> [w226]
          tunnel: w213 -> [w225]
          tunnel: w201 -> [w224]
          tunnel: w207 -> [w221]
          tunnel: [w223] -> w217
          tunnel: [w222] -> w216
          tunnel: [w221] -> w215
          tunnel: w200 -> [w220]
          tunnel: w199 -> [w219]
          tunnel: [w218] -> w198
          tunnel: [w262] -> w211
          tunnel: w217 -> [w264]
          tunnel: w216 -> [w263]
          tunnel: w215 -> [w261]
          tunnel: [w261] -> w206
          tunnel: [w260] -> w203
          tunnel: [w259] -> w197
          tunnel: w198 -> [w259]
          frame #0 {
            n59 = case shown="True" w221 {
              tunnel: w226 -> [w234 w253]
              tunnel: w225 -> [w232 w252]
              tunnel: [w231 w245] -> w222
              tunnel: w224 -> [_ _]
              tunnel: [w228 w244] -> w223
              tunnel: w220 -> [_ w239]
              tunnel: w219 -> [w227 w238]
              tunnel: [w227 w237] -> w218
              frame False {
                n60 = xnode "Invoke Method"("FPGA VI Reference In"=w234, "error in"=w232, "Number of Elements"=u32 0) -> ("FPGA VI Reference Out"=w230:refnum<k20>, "error out"=w229:errorcluster, "Elements Remaining"=w233:u32)  [unwired: 1 in, 1 out]
                n61 = xnode "Invoke Method"("FPGA VI Reference In"=w230, "error in"=w229, "Number of Elements"=w233) -> ("FPGA VI Reference Out"=w228:refnum<k20>, "error out"=w231:errorcluster)  [unwired: 1 in, 2 out]
              }
              frame True {
                n62 = xnode "Invoke Method"("FPGA VI Reference In"=w253, "error in"=w252, "Number of Elements"=u32 1024, "Timeout (ms)"=-1) -> ("FPGA VI Reference Out"=w247:refnum<k20>, "error out"=w246:errorcluster, "Data"=w249:fxp<+/-,12,12>[])  [unwired: 1 out]
                n63 = To Double Precision Float(number=w249) -> (double precision float=w240:dbl[])
                n64 = case shown="True" "Acrive Linearization" {
                  tunnel: w240 -> [_ w258]
                  tunnel: w239 -> [_ w257]
                  tunnel: w238 -> [w254 w256]
                  tunnel: [w254 w255] -> w237
                  frame False {
                  }
                  frame True {
                    n65 = RT FIFO Write(0:w257, 1:w258, 3:w256) -> (11:w255:errorcluster)  [unwired: 2 in, 3 out]
                  }
                }
                n66 = Split 1D Array(array=w240, index=512) -> (first subarray=→"First Signal (points) - Falling Triangular":dbl[], second subarray=→"Second Signal (points) - Rising Triangular":dbl[])
                n67 = xnode "Invoke Method"("FPGA VI Reference In"=w247, "error in"=w246, "Number of Elements"=u32 0) -> ("FPGA VI Reference Out"=w244:refnum<k20>, "error out"=w245:errorcluster)  [unwired: 1 in, 2 out]
              }
            }
          }
          frame #1 {
            n68 = case shown="True" w261 {
              tunnel: [w266 w269] -> w262
              tunnel: w264 -> [w265 w270]
              tunnel: w263 -> [w266 w268]
              tunnel: [w265 w267] -> w260
              frame False {
              }
              frame True {
                n69 = xnode "Read/Write Control"("FPGA VI Reference In"=w270, "error in"=w268, "snapshot"=FALSE) -> ("FPGA VI Reference Out"=w267:refnum<k20>, "error out"=w269:errorcluster)
              }
            }
          }
        }
        n70 = case shown="True" w210 {
          tunnel: w208 -> [w277 w298]
          tunnel: w209 -> [w274 w299]
          tunnel: [w273 w297] -> w212
          tunnel: w205 -> [_ w284]
          tunnel: w204 -> [_ w285]
          tunnel: w202 -> [_ w281]
          tunnel: w201 -> [_ w279]
          frame False {
            n71 = xnode "Invoke Method"("FPGA VI Reference In"=w277, "error in"=w274, "Number of Elements"=u32 0) -> ("FPGA VI Reference Out"=w275:refnum<k20>, "error out"=w272:errorcluster, "Elements Remaining"=w276:u32)  [unwired: 1 in, 1 out]
            n72 = xnode "Invoke Method"("FPGA VI Reference In"=w275, "error in"=w272, "Number of Elements"=w276) -> ("error out"=w273:errorcluster)  [unwired: 1 in, 3 out]
          }
          frame True {
            n73 = xnode "Invoke Method"("FPGA VI Reference In"=w298, "error in"=w299, "Number of Elements"=u32 512, "Timeout (ms)"=-1) -> ("FPGA VI Reference Out"=w295:refnum<k20>, "error out"=w296:errorcluster, "Data"=w301:fxp<+,44,44>[])  [unwired: 1 out]
            n74 = To Double Precision Float(number=w301) -> (double precision float=w300:dbl[])
            n75 = Square Root(x=w300) -> (sqrt(x)=w293:dbl[])
            n76 = Split 1D Array(array=w293, index=256) -> (first subarray=w291:dbl[], second subarray=w290:dbl[])
            "First FFT (bin)" <- w291
            "Second FFT (bin)" <- w290
            n77 = xnode "Invoke Method"("FPGA VI Reference In"=w295, "error in"=w296, "Number of Elements"=u32 0) -> ("error out"=w297:errorcluster)  [unwired: 1 in, 3 out]
            n78 = call "Distance-Velocity Calculation RT.vi"("First FFT"=w291, "Second FFT"=w290, "Windowing"=w281, "first FFT bin"=w284, "Sample Rate (S/s)"=w279, "last FFT bin"=w285) -> ("F_rise"=→"f_rise":dbl, "maxbin_firstFFT"=→"maxbin_firstFFT":i32, "maxbin_secondFFT"=→"maxbin_secondFFT":i32, "Distance (m)"=→"Distance (m)":dbl, "f_mean"=→"f_mean":dbl, "F_fall"=→"f_fall":dbl, "Velocity (m/s)"=→"Velocity (m/s)":dbl)  [unwired: 7 in]
          }
        }
      }
      frame #2 {
        n79 = case shown="True" w308 {
          tunnel: w305 -> [w311 w315]
          tunnel: [w311 w316] -> w304
          frame False {
          }
          frame True {
            n80 = Decrement(x="tieni premuto per") -> (x-1=w312:i32)
            n81 = Greater Or Equal?(x=w315, y=w312) -> (x >= y?=w314:bool)
            n82 = case shown="True" w314 {
              tunnel: w315 -> [w317 _]
              tunnel: [w318 0] -> w316
              frame False {
                n83 = Increment(x=w317) -> (x+1=w318:i32)
              }
              frame True {
                n84 = local write "Snapshot"(FALSE ("Snapshot")) -> ()
              }
            }
          }
        }
      }
    }
    n85 = node-c288() -> ()  [unwired: 1 in, 1 out]
  }
  n86 = node-c288(w32) -> ()  [unwired: 1 out]
  n87 = RT FIFO Delete(0:w12, 3:w11) -> (11:w10:errorcluster)  [unwired: 1 in]
  n88 = Merge Errors(w29, w30, w15, w10) -> (w13:errorcluster)
  n89 = flat-sequence {
    tunnel: w13 -> [w324]
    tunnel: w24 -> [w321]
    frame #0 {
      n90 = property on="stop" class="Bool (strict)"(error in=w324, "Value"=FALSE ("stop")) -> (error out=w323:errorcluster)  [unwired: 1 in, 1 out]
      n91 = xnode "Invoke Method"("FPGA VI Reference In"=w321, "error in"=w323) -> ("FPGA VI Reference Out"=w326:refnum<k20>, "error out"=w325:errorcluster)
      n92 = xnode "Invoke Method"("FPGA VI Reference In"=w326, "error in"=w325) -> ("FPGA VI Reference Out"=w327:refnum<k20>, "error out"=w328:errorcluster)
      n93 = xnode "Close FPGA VI Reference"("FPGA VI Reference In"=w327, "error in"=w328) -> ()  [unwired: 1 out]
    }
  }
